vi "getAO_chan_and_sampling.vi"(8 "error in (no error)":errorcluster, 11 "DAQ":refnum<class "DAQ.lvclass">[](array[class])) -> (0 "error out":errorcluster, 1 "sampling info":T1, 2 "Channels":T2[](array[typedef]), 3 "DAQ (AO)":refnum<class "DAQ.lvclass">[](array[class]))   [LabVIEW 2016, in "DAQ_Manager.lvclass"]
uses:
  DAQ_Manager.lvclass
  DAQ/DAQ.lvclass
  DAQ/Typedefs/PrivateEvents--DAQ.AI.Channels.ctl
  DAQ/Typedefs/DAQ_SamplingInfo.ctl
  DAQ/Typedefs/DAQ_Type.ctl
  DAQ/DAQ.lvclass/DAQ.ctl
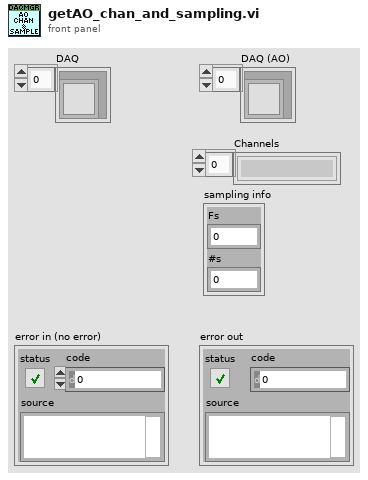
[diagram p1: front panel]
types:
  T1 = typedef "DAQ.lvclass/DAQ_SamplingInfo.ctl" = cluster{"Fs":dbl, "#s":i32}
  T2 = typedef "DAQ.lvclass/PrivateEvents--DAQ.AI.Channels.ctl" = string
  T3 = typedef "DAQ.lvclass/DAQ_Type.ctl" = enum16{"AI", "AO"}
  T4 = typedef "DAQ.lvclass/DAQ_Config.ctl" = cluster{"Channels":T2, "DAQ_Type":T3, "minimum value":dbl, "maximum value":dbl, "DAQ_SamplingInfo":T1, "DAQ_SamplingMode":T5}
  T5 = typedef "DAQ.lvclass/DAQ_SamplingMode.ctl" = enum16{"Continuous", "Finite"}
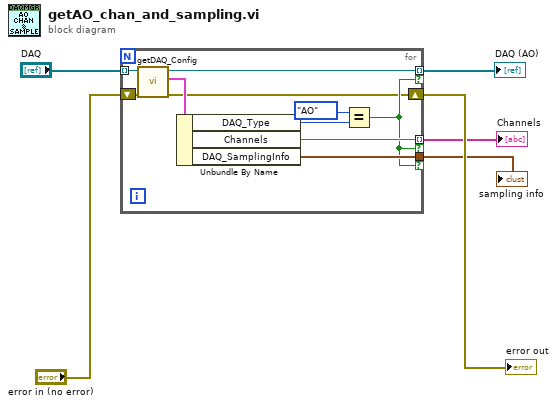
[diagram p0: block diagram]
diagram:
  n1 = for {
    tunnel: "DAQ" -> [w16] mode=indexing
    tunnel: [w14] -> w6 mode=indexing if=w9
    shift-right: [w7] -> w3
    shift-left: "error in (no error)" -> [w15]
    tunnel: [w13] -> w2 mode=indexing if=w9
    tunnel: [w12] -> w1 if=w9
    n2 = call "getDAQ_Config.vi"("error in (no error)"=w15, "DAQ in"=w16) -> ("error out"=w7:errorcluster, "DAQ_Config"=w8:T4, "DAQ out"=w14:refnum<class "DAQ.lvclass">)  [unwired: 7 in]
    n3 = Unbundle By Name(w8) -> ("DAQ_Type"=w10:T3, "Channels"=w13:T2, "DAQ_SamplingInfo"=w12:T1)
    n4 = Equal?(x=DAQ_Type."AO" ("DAQType"), y=w10) -> (x = y?=w9:bool)
  }
  "error out" <- w3
  "DAQ (AO)" <- w6
  "Channels" <- w2
  "sampling info" <- w1
